vi "未命名 3.vi"(1 "数值in":dbl) -> (0 "数值out":dbl)   [LabVIEW 2018]
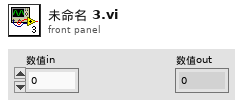
[diagram p1: front panel]
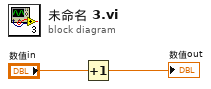
[diagram p0: block diagram]
diagram:
  n1 = Increment(x="数值in") -> (x+1=→"数值out":dbl)
